vi "Path_HDH ProjectBuilder Folder.vi"() -> (3 "HDH\\ProjectBuilder path":path)   [LabVIEW 2020, in "ProjectBuilder.lvlib"]
uses:
  PPL/HDH.ClassLoader.lvlibp/1abvi3w/vi.lib/Utility/sysdir.llb/HDH.ClassLoader_System Directory Type.ctl
  ProjectBuilder.lvlib
  PPL/HDH.ClassLoader.lvlibp
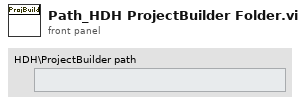
[diagram p1: front panel]
types:
  T1 = typedef "HDH.ClassLoader.lvlibp/HDH.ClassLoader_System Directory Type.ctl" = i32
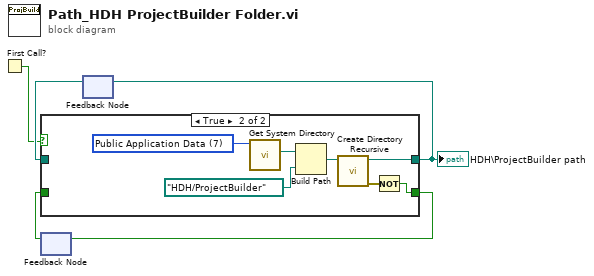
[diagram p0: block diagram]
diagram:
  n1 = First Call?() -> (First Call?: T/F=w1:bool)
  n2 = feedback #1() -> (w4:bool)  [unwired: 1 in]
  n3 = feedback #2() -> (w2:path)  [unwired: 1 in]
  n4 = case shown="True" w1 {
    tunnel: [w7 w10] -> w5
    tunnel: [w6 w8] -> w3
    tunnel: w2 -> [w7 _]
    tunnel: w4 -> [w6 _]
    frame False {
    }
    frame True {
      w14 = T1 7 items=["User Home"=0, "User Desktop"=1, "User Documents"=2, "User Application Data"=3, "User Preferences"=4, "User Temporary"=5, "Public Documents"=6, "Public Application Data"=7, "Public Preferences"=8, "Public Cache"=13, "System Core Libraries"=9, "System Installed Libraries"=10, "Application Files"=11, "Boot Volume Root"=12] ("system directory type")
      n5 = call <vilib>:"Get System Directory.vi"("system directory type"=w14) -> ("system directory"=w12:path)  [unwired: 10 in]
      n6 = Build Path(base path=w12, name or relative path=path "HDH/ProjectBuilder") -> (appended path=w11:path)
      n7 = call <vilib>:"Create Directory Recursive.vi"("directory"=w11) -> ("error out"=w9:errorcluster, "directory copy"=w10:path)  [unwired: 4 in, 1 out]
      n8 = Not(x=w9) -> (.not. x?=w8:bool)
    }
  }
  "HDH\\ProjectBuilder path" <- w5
  n9 = feedback-in #1(w3) -> ()
  n10 = feedback-in #2(w5) -> ()
